vi "cluster_from_settings_ini_file.vi"(8 "error in (no error)":errorcluster, 11 "containerIn":variant) -> (0 "error out":errorcluster, 3 "dataValue":variant)   [LabVIEW 2015, in "ini_work_Library.lvlib"]
doc: "Read keys from data/settings.ini file and fill cluster elements\n\n\nCreated by Artem Shevelev\nshevelev.pro\nartem@shevelev.pro\nLabVIEW Portal: https://labviewportal.org/memberlist.php?mode=viewprofile&u=2340"
uses:
  ini_work_Library.lvlib
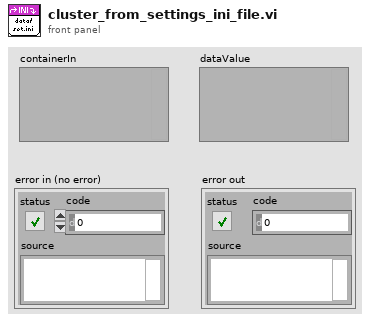
[diagram p1: front panel]
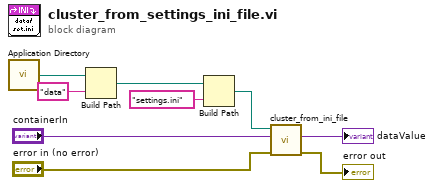
[diagram p0: block diagram]
diagram:
  n1 = call <vilib>:"Application Directory.vi"() -> ("Application Directory"=w1:path)
  n2 = Build Path(base path=w1, name or relative path="data") -> (appended path=w4:path)
  n3 = Build Path(base path=w4, name or relative path="settings.ini") -> (appended path=w5:path)
  n4 = call "cluster_from_ini_file.vi"("error in (no error)"="error in (no error)", "dataType"="containerIn", "iniFilePath"=w5) -> ("error out"=→"error out":errorcluster, "dataValue"=→"dataValue":variant)  [unwired: 7 in]
